vi "Get Name of Shared Variable for a Channel.vi"(9 "Channel Number":i32, 10 "Module Name":string, 11 "Module Position":string) -> (3 "Shared Variable Name":string)   [LabVIEW 2017, in "DTACQ - Network Enabled Device Driver.lvlib"]
uses:
  DTACQ - Network Enabled Device Driver.lvlib
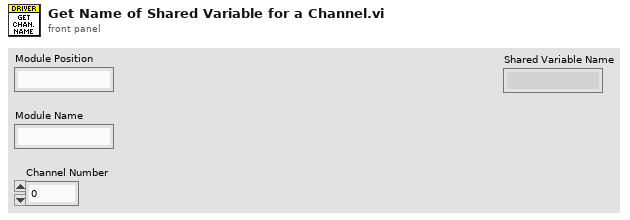
[diagram p1: front panel]
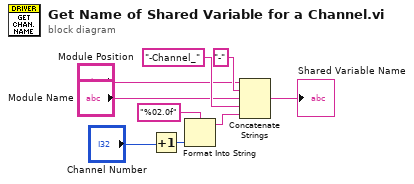
[diagram p0: block diagram]
diagram:
  n1 = Increment(x="Channel Number") -> (x+1=w8:i32)
  n2 = Format Into String(format string="%02.0f", w8) -> (resulting string=w9:string)  [unwired: 2 in, 1 out]
  n3 = Concatenate Strings("Module Position", "-", "Module Name", "-Channel_", w9) -> (→"Shared Variable Name":string)
